vi "handleErrors.vi"(8 "error in (no error)":errorcluster, 11 "TcpServer in":refnum<class "TcpServer.lvclass">) -> (0 "error out":errorcluster, 3 "TcpServer out":refnum<class "TcpServer.lvclass">)   [LabVIEW 2018, in "TcpServerCmd.lvclass"]
doc: "This function calls the clearErrorAndSendExplanation.vi."
uses:
  TcpServerCmd.lvclass
  TcpServer/TcpServer.lvclass
  TcpServer/TcpServer.lvclass/TcpServer.ctl
  home/pcortes/github/ts_labview_tcp_json/src/TcpServerBase/TcpServerBase.lvclass
  TcpServerBase/TcpServerBase.lvclass
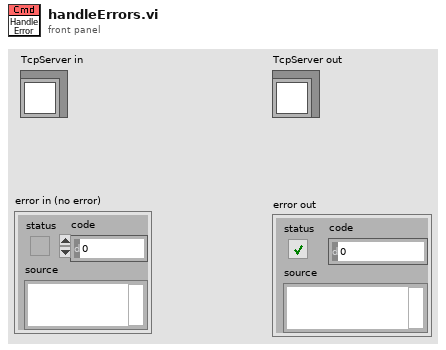
[diagram p1: front panel]
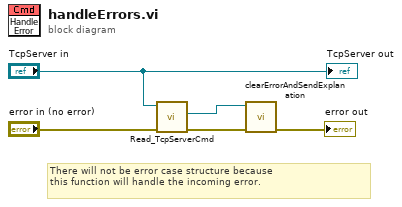
[diagram p0: block diagram]
diagram:
  # "There will not be error case structure because\nthis function will handle the incoming error."
  n1 = call "Read_TcpServerCmd.vi"("error in (no error)"="error in (no error)", "TcpServer in"="TcpServer in") -> ("error out"=w3:errorcluster, "TcpServerCmd.lvclass"=w2:refnum<class "TcpServerCmd.lvclass">)  [unwired: 7 in, 1 out]
  n2 = call "clearErrorAndSendExplanation.vi"("error in (no error)"=w3, "TcpServerBase in"=w2) -> ("error out"=→"error out":errorcluster)  [unwired: 8 in, 1 out]
  "TcpServer out" <- "TcpServer in"
